vi "XML Parse Zeitstempel.vi"(3 "Attribut Name":string, 7 "XML Response":string) -> (0 "Zeitstempel":timestamp, 1 "Zeit-Cluster":T1 caption="Ausgangs-Cluster", 2 "XML Response gekürzt":string)   [LabVIEW 2020, in "FT-IR.lvlib" / "TOOLweb Interface.lvlib" / "TOOLweb Interface Hilfs-VIs.lvlib"]
doc: "Sucht in dem XML-Poll-Response-String \"XML-Response\" den Eintrag mit dem Elementnamen \"Attribut Name\" und liefert dessen Wert als Zeitstempel und als Zeit-Cluster.\n\nDer Eintrag wird dann entfernt, damit eine weiteres Parser-VI am Ausgang \"XML Response gekürzt\" nicht wieder den ganzen String durchsuchen muss."
uses:
  TOOLweb Interface Hilfs-VIs.lvlib
  <vilib>/Utility/miscctls.llb/LVDateTimeRec.ctl
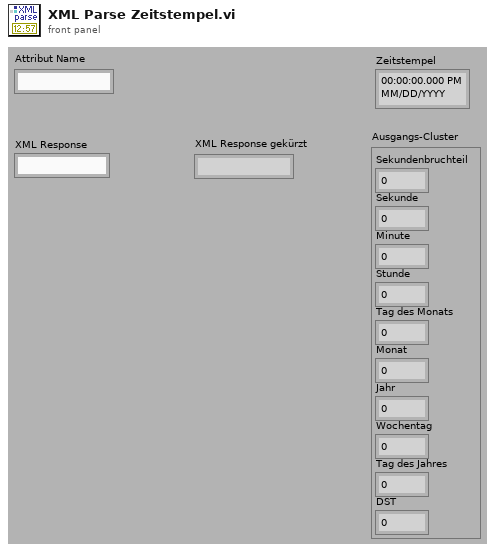
[diagram p1: front panel]
types:
  T1 = typedef "LVDateTimeRec.ctl" = cluster{"fractional second":dbl, "second":i32, "minute":i32, "hour":i32, "day of month":i32, "month":i32, "year":i32, "day of week":i32, "day of year":i32, "DST":i32}
  T2 = enum16{"YYYYMMDD HH:MM:SS", "[YYMMDD][HH:MM:SS]"}
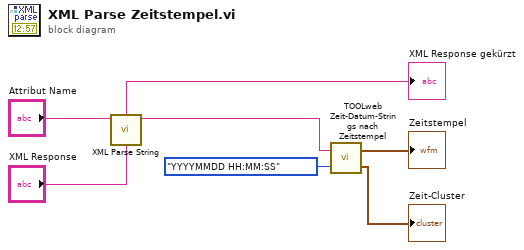
[diagram p0: block diagram]
diagram:
  n1 = call "XML Parse String.vi"("Attribut Name"="Attribut Name", "XML Response"="XML Response") -> ("Wert-String"=w4:string, "XML Response gekürzt"=→"XML Response gekürzt":string)  [unwired: 6 out]
  n2 = call "TOOLweb Zeit-Datum-Strings nach Zeitstempel.vi"("Format"=T2."YYYYMMDD HH:MM:SS", "Zeit/Datum-String"=w4) -> ("Zeit-Cluster"=→"Zeit-Cluster":T1, "Zeitstempel"=→"Zeitstempel":timestamp)
